vi "Drive Set.vi"() -> ()   [LabVIEW 2017]
uses:
  <vilib>/Rock Robotics/WPI/DriverStation/WPI_DriverStationRobotMode2.ctl
  Drive Control Type.ctl
  Drive Globals.vi
  Robot Global Data.vi
panel:
  out "error out 2":errorcluster
  out "error out":errorcluster
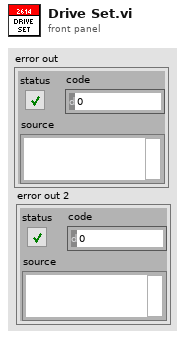
[diagram p1: front panel]
types:
  T1 = typedef "Drive Control Type.ctl" = enum16{"No_Op", "Basic Drive", "Time", "Heading", "RC_Speed", "Switch_Slots", "AutoTrack_Cube", "Speed Test", "Turn_Cube", "To_Cube", "Wait", "Distance_Slow", "Distance", "Distance_Ramp"}
  T2 = typedef "WPI_DriverStationRobotMode2.ctl" = enum16{"Autonomous Disabled", "Autonomous Enabled", "Teleop Disabled", "Teleop Enabled", "Disconnected", "Finish", "Test Disabled", "Test Enabled", "Emergency Stopped"}
  T3 = typedef "Drive Notifier.ctl" = cluster{"Drive Control Type":T1, "Throttle":dbl, "Twist":dbl, "Step":i32, "High Gear":bool, "Parameter 1":dbl, "Parameter 2":dbl, "Parameter 3":dbl, "Drive Notifier":refnum<notifier>, "AutoTrack":bool}
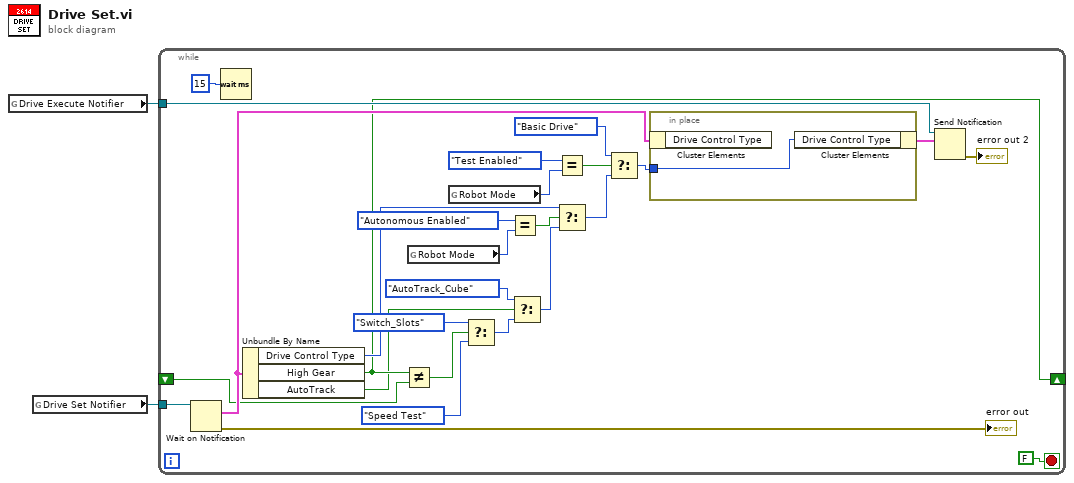
[diagram p0: block diagram]
diagram:
  n1 = global read "Drive Globals.vi" "Drive Execute Notifier"() -> (w1:refnum<notifier>)
  n2 = global read "Drive Globals.vi" "Drive Set Notifier"() -> (w2:refnum<notifier>)
  n3 = while {
    tunnel: w2 -> [w26]
    tunnel: w1 -> [w25]
    shift-right: [w12] -> _
    shift-left: _ -> [w13]
    stop <- FALSE stop-if-true
    n4 = Wait on Notification(notifier=w26) -> (notification=w24:T3, error out=→"error out":errorcluster)  [unwired: 3 in, 2 out]
    n5 = Wait (ms)(milliseconds to wait=u32 15) -> ()  [unwired: 1 out]
    n6 = Unbundle By Name(w24) -> ("Drive Control Type"=w20:T1, "High Gear"=w12:bool, "AutoTrack"=w6:bool)
    n7 = Not Equal?(x=w12, y=w13) -> (x != y?=w11:bool)
    n8 = global read "Robot Global Data.vi" "Robot Mode"() -> (w22:T2)
    n9 = global read "Robot Global Data.vi" "Robot Mode"() -> (w18:T2)
    n10 = Select(t=Drive_Control_Type."Switch_Slots", s=w11, f=Drive_Control_Type."Speed Test") -> (s? t:f=w8:T1)
    n11 = Equal?(x=WPI_DriverStationRobotMode2."Autonomous Enabled", y=w22) -> (x = y?=w23:bool)
    n12 = Select(t=Drive_Control_Type."AutoTrack_Cube", s=w6, f=w8) -> (s? t:f=w7:T1)
    n13 = Equal?(x=WPI_DriverStationRobotMode2."Test Enabled", y=w18) -> (x = y?=w15:bool)
    n14 = Select(t=w20, s=w23, f=w7) -> (s? t:f=w17:T1)
    n15 = Select(t=Drive_Control_Type."Basic Drive", s=w15, f=w17) -> (s? t:f=w16:T1)
    n16 = in-place {
      in-place-border: w16 -> [w30]
      n17 = in-place-cluster #1(w24) -> ()  [unwired: 1 out]
      n18 = in-place-cluster #1("Drive Control Type"=w30) -> (w27:T3)
    }
    n19 = Send Notification(notification=w27, notifier=w25) -> (error out=→"error out 2":errorcluster)  [unwired: 1 in, 1 out]
  }
